vi "Entry.vi"(8 "error in (no error)":errorcluster, 11 "New State":refnum<class "UC_Idle.lvclass">) -> (0 "error out":errorcluster, 3 "State out":refnum<class "UC_Idle.lvclass">)   [LabVIEW 2025, in "User_Console.lvlib" / "UC_Idle.lvclass"]
doc: "This is an abstract method. Override this method to define the behavior when you enter the state."
uses:
  UC_Idle.lvclass
  UC_Idle.lvclass/UC_Idle.ctl
  User_Console/User_Console.lvclass
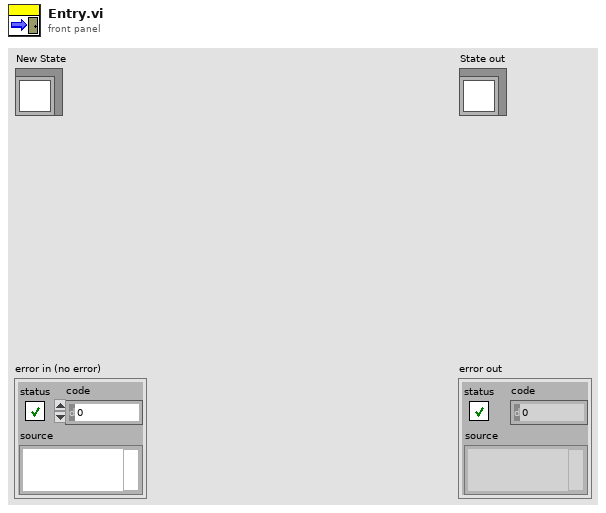
[diagram p1: front panel]
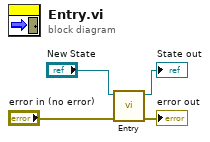
[diagram p0: block diagram]
diagram:
  n1 = call-parent "Entry.vi"("error in (no error)"="error in (no error)", "New State"="New State") -> ("error out"=→"error out":errorcluster, "State out"=→"State out":refnum<class "UC_Idle.lvclass">)  [unwired: 8 in]
